vi "TC01_Temp_FEEDBACK.vi"() -> ()   [LabVIEW 2022 SP3]
uses:
  <vilib>/Utility/file.llb/Write To Spreadsheet File (DBL).vi
panel:
  in  "Path":path=path "D:/Labview Programs/HIFU_TEMP"
  in  "Filename":string="Filename"
  out "Numeric":u32
  out "Waveform Chart":dynamicdata(graph)
  out "data":dbl
  out "error out":errorcluster
  in  "stop (F)":bool
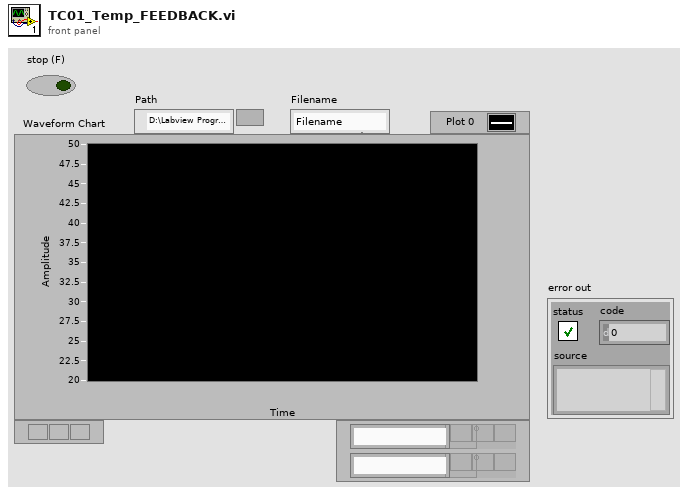
[diagram p1: front panel]
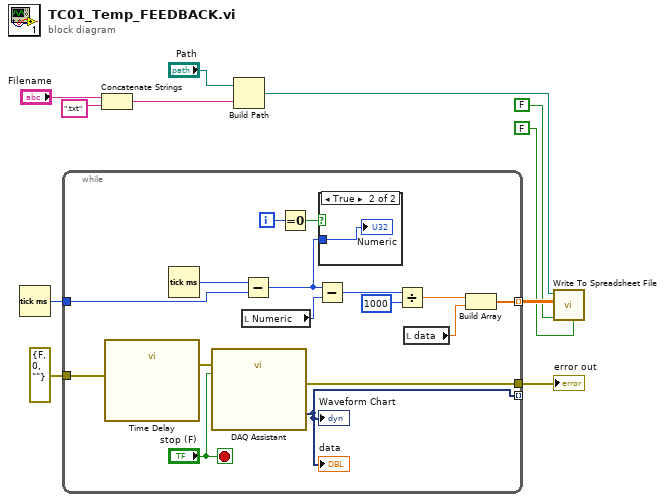
[diagram p0: block diagram]
diagram:
  n1 = Tick Count (ms)() -> (millisecond timer value=w9:u32)
  n2 = while {
    tunnel: [w17] -> _ mode=indexing
    tunnel: errorcluster {"status"=FALSE, "code"=0, "source"=""} ("error in") -> [w25]
    tunnel: [w27] -> w10
    tunnel: w9 -> [w23]
    tunnel: [w15] -> w8 mode=indexing
    i -> [w21]
    stop <- "stop (F)" stop-if-true
    n3 = call "Time Delay"("error in (no error)"=w25) -> ("error out"=w24:errorcluster)  [unwired: 10 in]
    n4 = Tick Count (ms)() -> (millisecond timer value=w22:u32)
    n5 = call "DAQ Assistant"("error in"=w24, "stop (F)"="stop (F)") -> ("data"=w17:dynamicdata, "error out"=w27:errorcluster)  [unwired: 15 in, 1 out]
    "data" <- w17
    "Waveform Chart" <- w17
    n6 = local read "Numeric"() -> (w18:u32)
    n7 = Subtract(x=w22, y=w23) -> (x-y=w19:u32)
    n8 = Equal To 0?(x=w21) -> (x = 0?=w20:bool)
    n9 = Subtract(x=w19, y=w18) -> (x-y=w14:u32)
    n10 = case shown="True" w20 {
      tunnel: w19 -> [_ w28]
      frame False {
      }
      frame True {
        "Numeric" <- w28
      }
    }
    n11 = Divide(x=w14, y=u32 1000) -> (x/y=w13:dbl)
    n12 = local read "data"() -> (w16:dbl)
    n13 = Build Array(w13, w16) -> (w15:dbl[])
  }
  "error out" <- w10
  n14 = Concatenate Strings("Filename", ".txt" ("string")) -> (w3:string)
  n15 = Build Path(base path="Path", name or relative path=w3) -> (appended path=w6:path)
  n16 = call-poly <vilib>:"Write To Spreadsheet File.vi"("transpose? (no:F)"=FALSE, "append to file? (new file:F)"=FALSE, "2D data"=w8, "file path (dialog if empty)"=w6) -> ()  [unwired: 4 in, 1 out]
